vi "StartAlbumAcq TimeLoop.vi"() -> ()   [LabVIEW 2019]
uses:
  Settings/System Running Settings.ctl
  Support/Hardware Configuration.ctl
  Support/Camera Configuration.ctl
  C:/RM21-MMicrosopeSource/HardwareAdapter/Camera/Dependencies/PVCamNET.dll
  Dependencies/PVCamNET.dll
  <vilib>/vision/Image Controls.llb/IMAQ Image.ctl
  C:/RM21-MMicrosopeSource/HardwareAdapter/Lasers/Dependencies/Oxxius_Boxx.dll
  Lasers/Dependencies/Oxxius_Boxx.dll
  Logging/Logging Configuration.ctl
  Controls/DeviceStatusCtl.ctl
  Controls/CallBack Refs.ctl
  <vilib>/Platform/TimedLoop/XDataNode/timing_clust.ctl
  <vilib>/Platform/TimedLoop/XDataNode/nitl_modes.ctl
  <vilib>/Platform/TimedLoop/XDataNode/wakeup.ctl
  <vilib>/Platform/TimedLoop/XDataNode/XDataNode.xnode
  <vilib>/Platform/TimedLoop/XDataNode/XDNodeRunTimeDep.lvlib
  Logging/Logging.lvlib
  Settings/Settings.lvlib
panel:
  in  "AcquisitionMode":i32
  in  "FramesToCapture":u16=1
  in  "Period":i64=1000
  in  "Exposure":u32=1000
  in  "TotalFrames":i32=3
  out "Busy":bool=TRUE
  out "Numeric":i32
  out "millisecond timer value":u32
  out "RawImage":T1(plugin-control)
  in  "Config In":T2 {"Hardware Configuration"."Lasers Configuration"."SettingValues"."785 Power" format="%.1f"; "Hardware Configuration"."Lasers Configuration"."SettingValues"."647 Power" format="%.1f"; "Hardware Configuration"."Lasers Configuration"."SettingValues"."561 Power" format="%.1f"}
  out "Config Out":T2 {"Hardware Configuration"."Lasers Configuration"."SettingValues"."785 Power" format="%.1f"; "Hardware Configuration"."Lasers Configuration"."SettingValues"."647 Power" format="%.1f"; "Hardware Configuration"."Lasers Configuration"."SettingValues"."561 Power" format="%.1f"}
  in  "error in (no error)":errorcluster
  out "error out":errorcluster
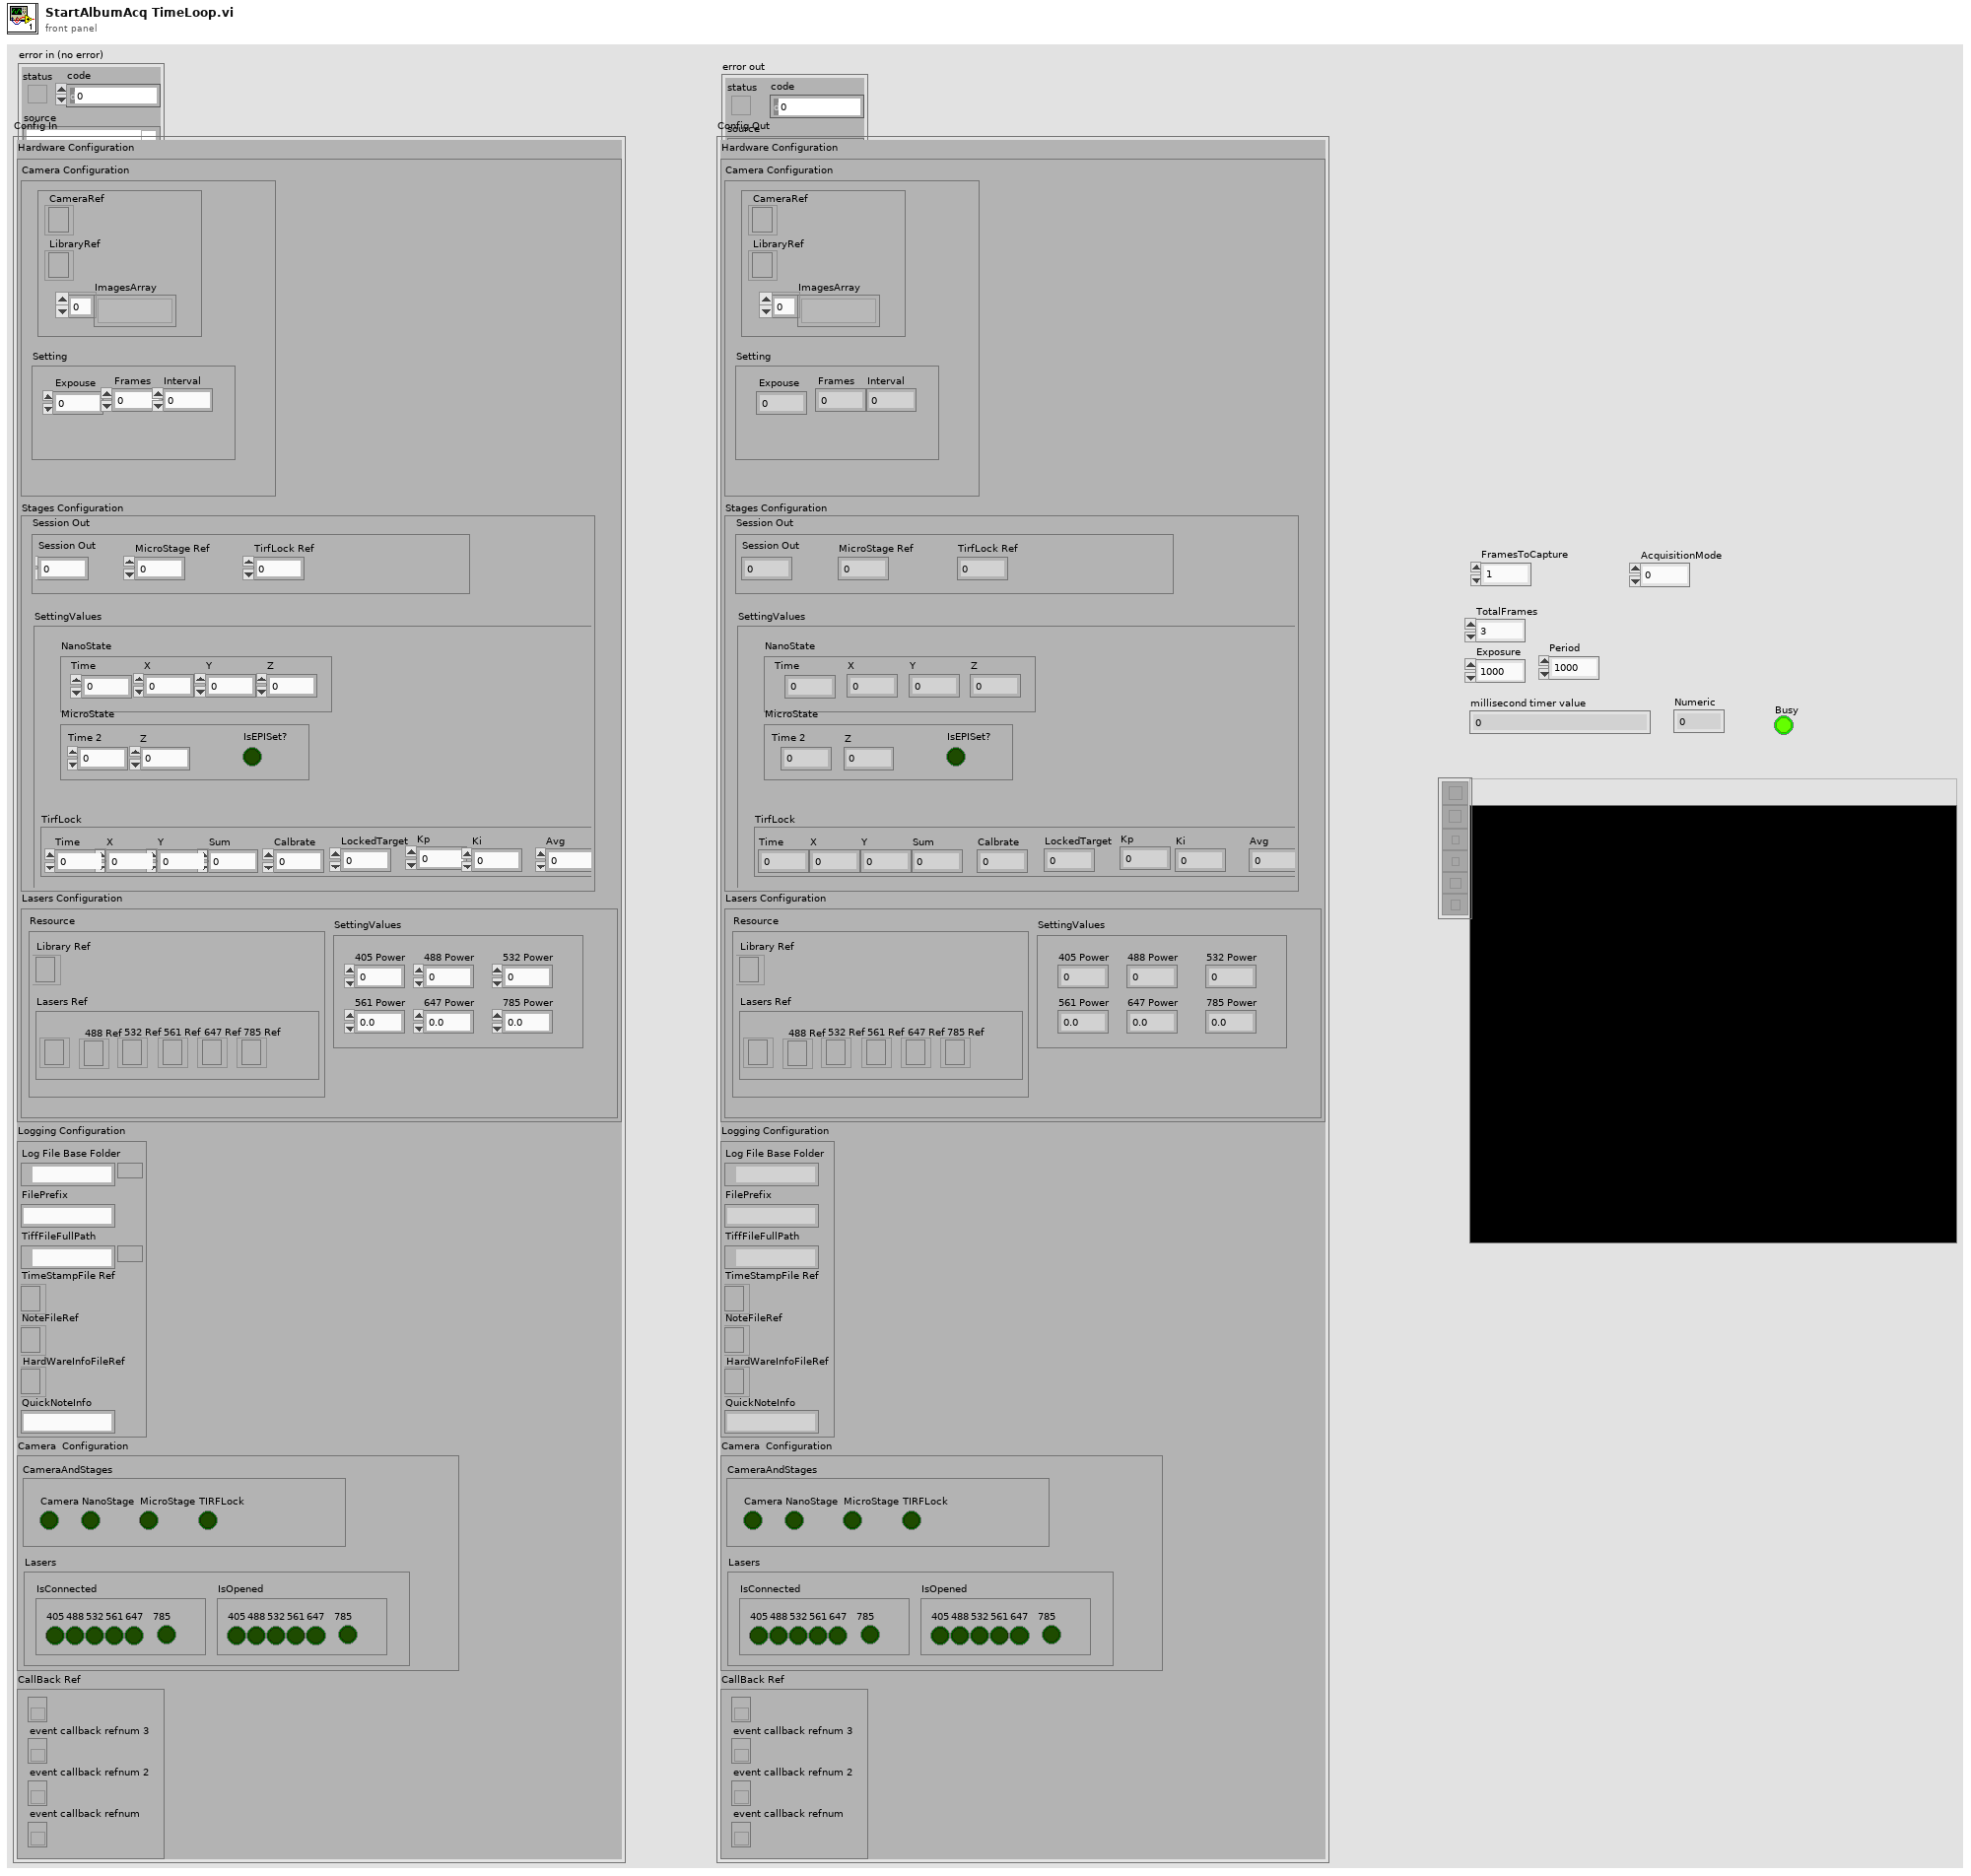
[diagram p1: front panel]
types:
  T1 = typedef "IMAQ Image.ctl" = refnum<image>
  T2 = typedef "Settings.lvlib/System Running Settings.ctl" = cluster{"Hardware Configuration":T3, "Logging Configuration":T5, "HardWare Status":cluster{"CameraAndStages":T6, "Lasers":cluster{"IsConnected":cluster{"405":bool, "488":bool, "532":bool, "561":bool, "647":bool, "785":bool}, "IsOpened":cluster{"405":bool, "488":bool, "532":bool, "561":bool, "647":bool, "785":bool}}}, "CallBack Ref":T7}
  T3 = typedef "Hardware Configuration.ctl" = cluster{"Camera Configuration":T4, "Stages Configuration":cluster{"Resource":cluster{"NanoStage Ref":i32, "MicroStage Ref":i32, "TirfLock Ref":i32}, "SettingValues":cluster{"NanoState":cluster{"Time":dbl, "X":dbl, "Y":dbl, "Z":dbl}, "MicroState":cluster{"Time 2":dbl, "Z":dbl, "IsEPISet?":bool}, "TirfLock":cluster{"Time":dbl, "X":dbl, "Y":dbl, "Sum":dbl, "Calbrate":dbl, "LockedTarget":dbl, "Kp":dbl, "Ki":dbl, "Avg":dbl}}}, "Lasers Configuration":cluster{"SettingValues":cluster{"405 Power":sgl, "488 Power":sgl, "532 Power":sgl, "561 Power":sgl, "647 Power":sgl, "785 Power":sgl}, "Resource":cluster{"Library Ref":refnum<k24>, "Lasers Ref":cluster{"405 Ref":refnum<k24>, "488 Ref":refnum<k24>, "532 Ref":refnum<k24>, "561 Ref":refnum<k24>, "647 Ref":refnum<k24>, "785 Ref":refnum<k24>}}}}
  T4 = typedef "Camera Configuration.ctl" = cluster{"Setting":cluster{"Expouse":dbl, "Frames":dbl, "Interval":dbl}, "Resource":cluster{"CameraRef":refnum<k24>, "LibraryRef":refnum<k24>, "ImagesArray":T1[]}}
  T5 = typedef "Logging.lvlib/Logging Configuration.ctl" = cluster{"Log File Base Folder":path, "FilePrefix":string, "TiffFileFullPath":path, "TimeStampFile Ref":refnum<file>, "NoteFileRef":refnum<file>, "HardWareInfoFileRef":refnum<file>, "QuickNoteInfo":string}
  T6 = typedef "DeviceStatusCtl.ctl" = cluster{"Camera":bool, "NanoStage":bool, "MicroStage":bool, "TIRFLock":bool}
  T7 = typedef "CallBack Refs.ctl" = cluster{"event callback refnum":refnum<k27>, "event callback refnum 2":refnum<k27>, "event callback refnum 3":refnum<k27>, "event callback refnum 4":refnum<k27>}
  T8 = typedef "Image Type" = u32
  T9 = typedef "XDNodeRunTimeDep.lvlib/timing_clust.ctl" = cluster{"Expected End [f-1]":u64, "Actual End [f-1]":u64, "Finished Late? [f-1]":bool, "Expected End [i-1]":u64, "Actual End [i-1]":u64, "Finished Late? [i-1]":bool, "Expected Start [i]":u64, "Actual Start [i]":u64, "Expected Start [f]":u64, "Actual Start [f]":u64, "Source Name":string, "Structure Name":string, "Period":i64, "Deadline":i64, "Offset":i64, "Start":i64, "Priority":i32, "Timeout":i32, "Mode":T10, "Wakeup Reason":T11, "Error":errorcluster, "Source Type":string, "Secondary Source Type":string, "Global End Time":u64, "Global Start Time":u64, "Frame Duration":u64, "Iteration Duration":u64, "Assigned CPU":i32, "I/O Scan Engine Mode":u32}
  T10 = typedef "XDNodeRunTimeDep.lvlib/nitl_modes.ctl" = enum32{"No Change", "Process missed periods, maintain original phase", "Discard missed periods, maintain original phase", "Process missed periods, ignore original phase", "Discard missed periods, ignore original phase"}
  T11 = typedef "XDNodeRunTimeDep.lvlib/wakeup.ctl" = enum32{"Normal", "Aborted", "Asynchronous wakeup", "Timing source error", "Timed loop error", "Timeout"}
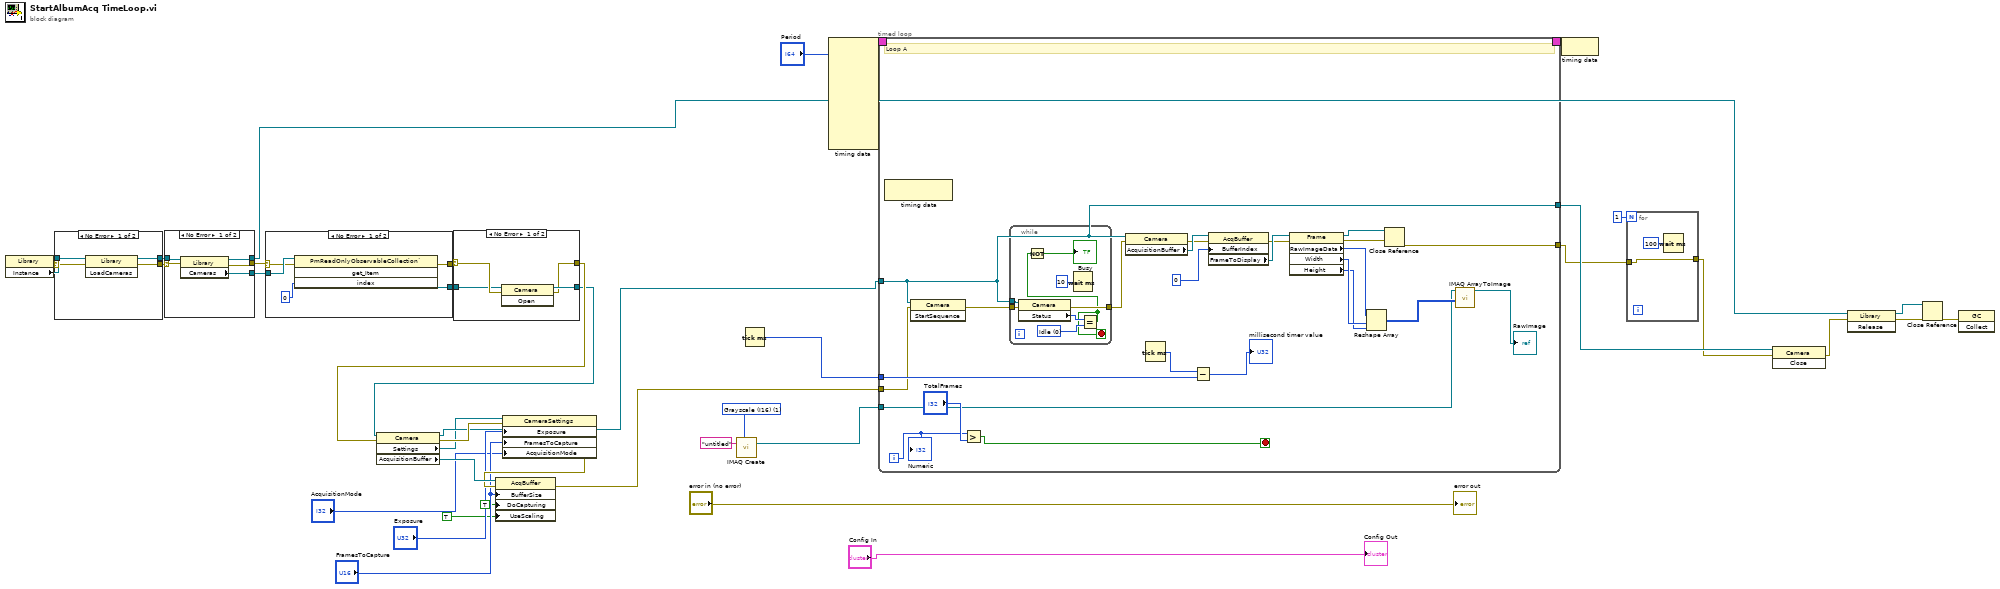
[diagram p0: block diagram]
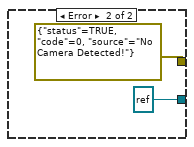
[diagram p2: hidden frame]
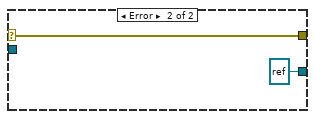
[diagram p3: hidden frame]
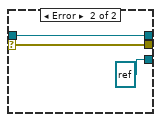
[diagram p4: hidden frame]
diagram:
  w35 = T8 1 items=["Grayscale (U8)", "Grayscale (I16)", "Grayscale (SGL)", "Complex (CSG)", "RGB (U32)", "HSL (U32)", "RGB (U64)", "Grayscale (U16)"] ("Image Type")
  n1 = property class="Library"() -> (error out=w32:errorcluster, "Instance"=w29:refnum<k24>)  [unwired: 2 in, 1 out]
  n2 = case shown="No Error" w32 {
    selector: w32 -> [w41 w45]
    tunnel: [w42 w45] -> w30
    tunnel: [w43 w44] -> w31
    tunnel: w29 -> [w40 w44]
    frame No Error {
      n3 = invoke class="Library" method="LoadCameras"(reference=w40, error in=w41) -> (reference out=w43:refnum<k24>, error out=w42:errorcluster)  [unwired: 1 in, 1 out]
    }
    frame Error {
    }
  }
  n4 = case shown="No Error" w30 {
    selector: w30 -> [w50 w53]
    tunnel: [w47 w53] -> w26
    tunnel: w31 -> [w49 w52]
    tunnel: [w48 w52] -> w14
    tunnel: [w46 refnum<k24> refnum ("Cameras")] -> w28
    frame No Error {
      n5 = property class="Library"(reference=w49, error in=w50) -> (reference out=w48:refnum<k24>, error out=w47:errorcluster, "Cameras"=w46:refnum<k24>)
    }
    frame Error {
    }
  }
  n6 = case shown="No Error" w26 {
    selector: w26 -> [w55 w60]
    tunnel: w28 -> [w58 _]
    tunnel: [w56 refnum<k24> refnum ("get_Item")] -> w27
    tunnel: [w54 w60] -> w25
    frame No Error {
      n7 = invoke class="PmReadOnlyObservableCollection`" method="get_Item"(reference=w58, error in=w55, "index"=0) -> (error out=w54:errorcluster, "get_Item"=w56:refnum<k24>)  [unwired: 1 in, 2 out]
    }
    frame Error {
    }
  }
  n8 = case shown="No Error" w25 {
    selector: w25 -> [w63 _]
    tunnel: [w62 errorcluster {"status"=TRUE, "code"=0, "source"="No Camera Detected!"} ("error out")] -> w8
    tunnel: w27 -> [w61 _]
    tunnel: [w64 refnum<k24> refnum ("get_Item")] -> w3
    frame No Error {
      n9 = invoke class="Camera" method="Open"(reference=w61, error in=w63) -> (reference out=w64:refnum<k24>, error out=w62:errorcluster)  [unwired: 1 in, 1 out]
    }
    frame Error {
    }
  }
  n10 = property class="Camera"(reference=w3, error in=w8) -> (reference out=w9:refnum<k24>, error out=w24:errorcluster, "Settings"=w1:refnum<k24>, "AcquisitionBuffer"=w23:refnum<k24>)
  n11 = property class="CameraSettings"(reference=w1, error in=w24, "Exposure"="Exposure", "FramesToCapture"="FramesToCapture", "AcquisitionMode"="AcquisitionMode") -> (error out=w22:errorcluster)  [unwired: 1 out]
  n12 = property class="AcqBuffer"(reference=w23, error in=w22, "BufferSize"="FramesToCapture", "DoCapturing"=TRUE, "UseScaling"=TRUE) -> (error out=w12:errorcluster)  [unwired: 1 out]
  n13 = call "IMAQ Create"("Image Name"="untitled", "Image Type"=w35) -> ("New Image"=w33:T1)  [unwired: 3 in, 1 out]
  n14 = Tick Count (ms)() -> (millisecond timer value=w13:u32)
  n15 = node-c288("Period") -> (w39:T9)  [unwired: 9 in]
  n16 = timed-loop {
    timing-out: [_] -> w38
    timing: w39 -> [_]
    tunnel: w12 -> [w68]
    tunnel: w33 -> [w76]
    tunnel: w9 -> [w70]
    tunnel: [w70] -> w16
    tunnel: w13 -> [w74]
    tunnel: [w67] -> w6
    i -> [w88]
    stop <- w89 stop-if-true
    # "Loop A"
    n17 = node-c288() -> ()  [unwired: 1 in, 1 out]
    n18 = invoke class="Camera" method="StartSequence"(reference=w70, error in=w68) -> (error out=w69:errorcluster)  [unwired: 1 in, 2 out]
    n19 = Greater?(x=w88, y="TotalFrames") -> (0:w89:bool)
    n20 = while {
      tunnel: w70 -> [w96]
      tunnel: w69 -> [w95]
      tunnel: [w94] -> w71
      stop <- w91 stop-if-true
      w98 = 0 items=["Idle", "Capturing"] ("Status")
      n21 = property class="Camera"(reference=w96, error in=w95) -> (error out=w94:errorcluster, "Status"=w97:i32)  [unwired: 1 out]
      n22 = Wait (ms)(milliseconds to wait=u32 10) -> ()  [unwired: 1 out]
      n23 = Equal?(x=w97, y=w98) -> (x = y?=w91:bool)
      n24 = Not(x=w91) -> (.not. x?=→"Busy":bool)
    }
    n25 = property class="Camera"(reference=w70, error in=w71) -> (error out=w86:errorcluster, "AcquisitionBuffer"=w87:refnum<k24>)  [unwired: 1 out]
    n26 = Tick Count (ms)() -> (millisecond timer value=w73:u32)
    n27 = Subtract(x=w73, y=w74) -> (x-y=→"millisecond timer value":u32)
    n28 = property class="AcqBuffer"(reference=w87, error in=w86, "BufferIndex"=0) -> (error out=w84:errorcluster, "FrameToDisplay"=w85:refnum<k24>)  [unwired: 1 out]
    n29 = property class="Frame"(reference=w85, error in=w84) -> (reference out=w79:refnum<k24>, error out=w78:errorcluster, "RawImageData"=w83:i16[], "Width"=w82:u32, "Height"=w81:u32)
    n30 = Reshape Array "Reshape Array"(w83, w82, w81) -> (w80:i16[][])
    n31 = Close Reference(reference=w79, error in (no error)=w78) -> (error out=w67:errorcluster)
    n32 = call "IMAQ ArrayToImage"("Image Pixels (I16)"=w80, "Image"=w76) -> ("Image Out"=→"RawImage":T1)  [unwired: 8 in, 1 out]
    "Numeric" <- w88
  }
  n33 = node-c288(w38) -> ()
  n34 = for {
    N: 1 -> [_]
    tunnel: w6 -> [w101]
    tunnel: [w101] -> w4
    n35 = Wait (ms)(milliseconds to wait=u32 100) -> ()  [unwired: 1 out]
  }
  n36 = invoke class="Camera" method="Close"(reference=w16, error in=w4) -> (error out=w15:errorcluster)  [unwired: 1 in, 2 out]
  n37 = invoke class="Library" method="Release"(reference=w14, error in=w15) -> (reference out=w17:refnum<k24>, error out=w19:errorcluster)  [unwired: 1 in, 1 out]
  n38 = Close Reference(reference=w17, error in (no error)=w19) -> (error out=w18:errorcluster)
  n39 = invoke class="GC" method="Collect"(error in=w18) -> ()  [unwired: 2 in, 3 out]
  "error out" <- "error in (no error)"
  "Config Out" <- "Config In"
